vi "Email Handler (PC).vi"() -> ()   [LabVIEW 2019]
uses:
  Controls/Alarm Config.ctl
  Controls/Alarm Definition.ctl
  Controls/Alarm Profile Config.ctl
panel:
  in  "Boolean":bool
  out "Tab Control":enum32{"Page 1", "Page 2"}(tab)
  in  "Email To:":string
  out "Unsent Emails":i32
  in  "Script Path":path=path "C:/Projects/Alarm Email Handler/Executable/Script/gmail_script.py"
  in  "Path to Python.exe":path=path "C:/Python35-32/python.exe"
  # "Keep Running\nand Minimized"
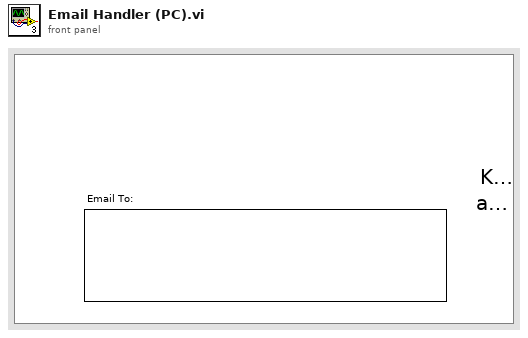
[diagram p1: front panel]
types:
  T1 = cluster{"ArmedAddresses":i32[], "Tracker":i32, "Armed":bool, "Email To:":string, "Alarm":bool, "Unsent Emails":i32, "IP to Check":i32, "Email Data":string[], "Email Config Path":path}
  T2 = enum16{"open", "replace", "create", "open or create", "replace or create", "replace or create with confirmation"}
  T3 = typedef "Alarm Config.ctl" = cluster{"Alarms:":T4[], "Profile Sync:":T5}
  T4 = typedef "Alarm Definition.ctl" = cluster{"Description:":string, "Enabled:":bool, "Data Index:":i32, "Data Type:":string, "Low Limit:":dbl, "High Limit:":dbl, "Trip Time:":u32, "Profile Sync:":bool}
  T5 = typedef "Alarm Profile Config.ctl" = cluster{"Trip Time:":u32, "Consecutive Trips:":i32}
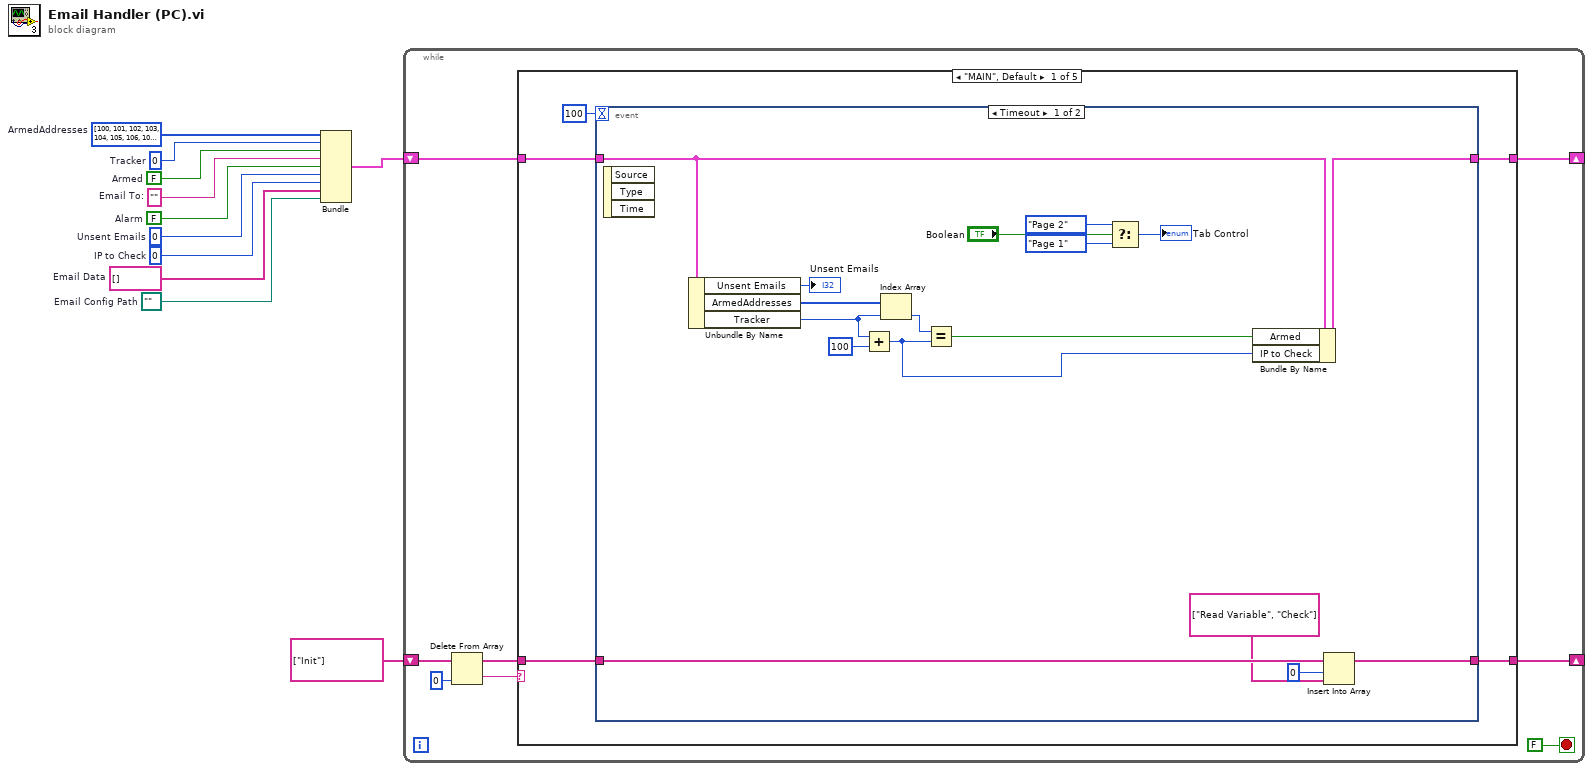
[diagram p0: block diagram]
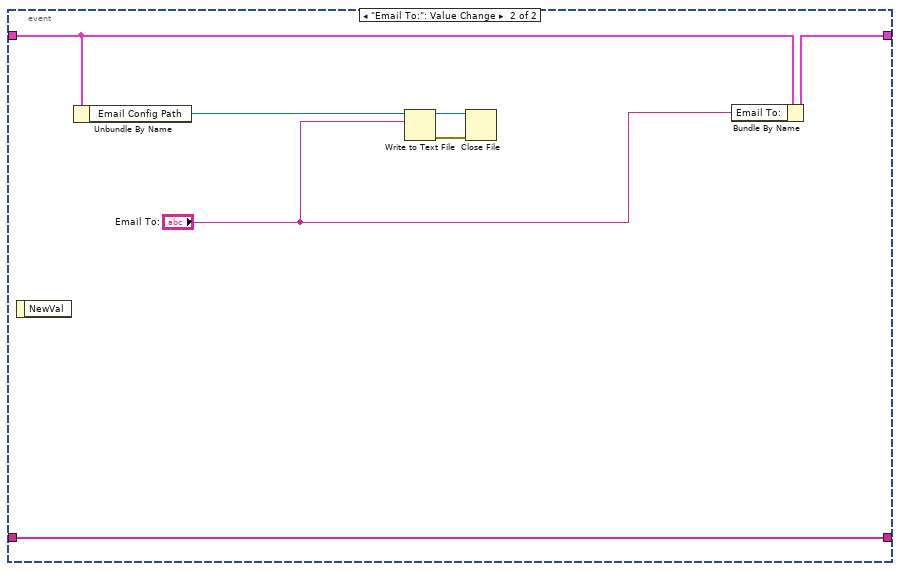
[diagram p2: hidden frame]
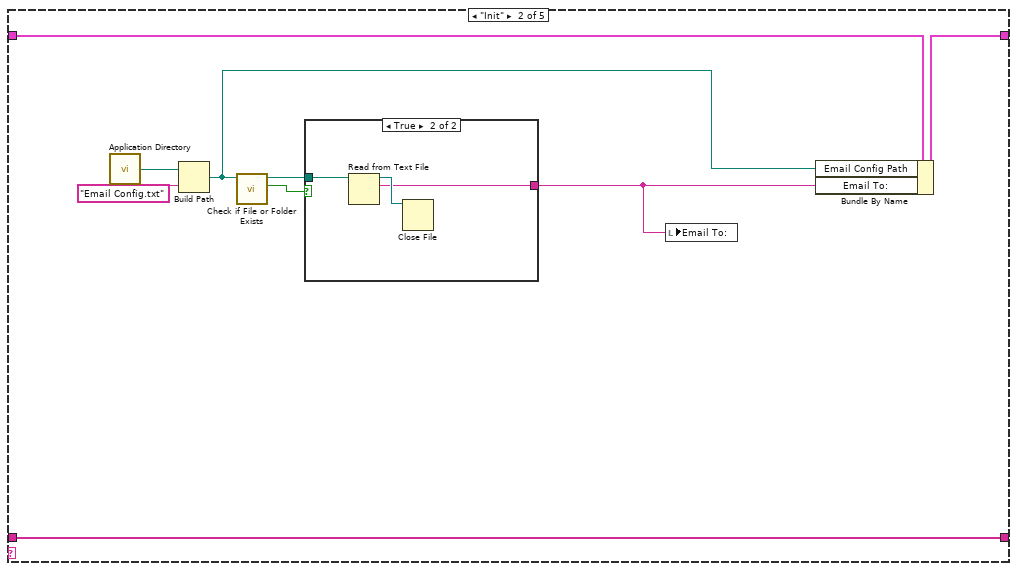
[diagram p3: hidden frame]
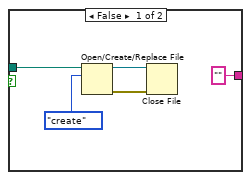
[diagram p4: hidden frame]
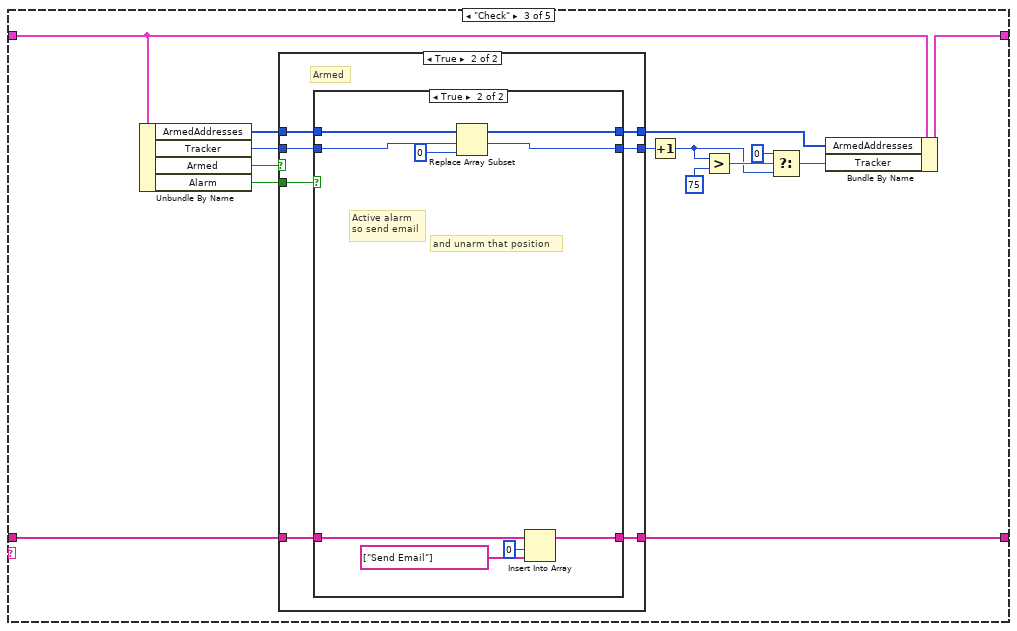
[diagram p5: hidden frame]
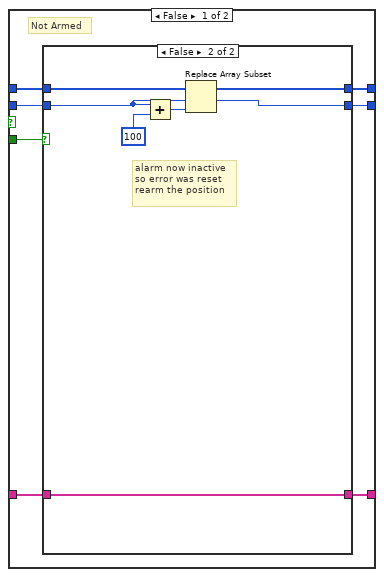
[diagram p6: hidden frame]
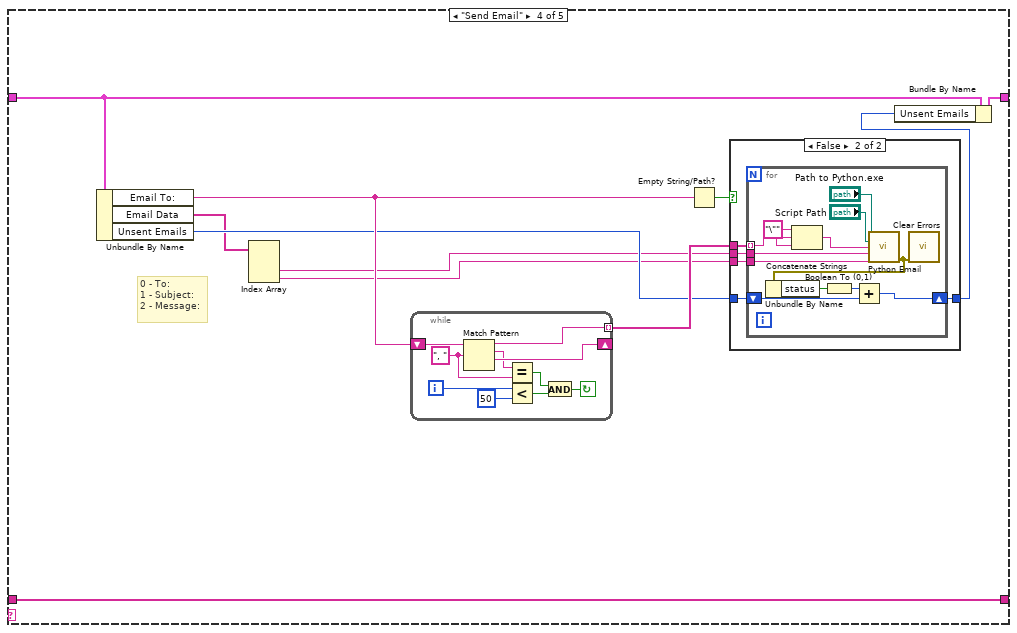
[diagram p9: hidden frame]
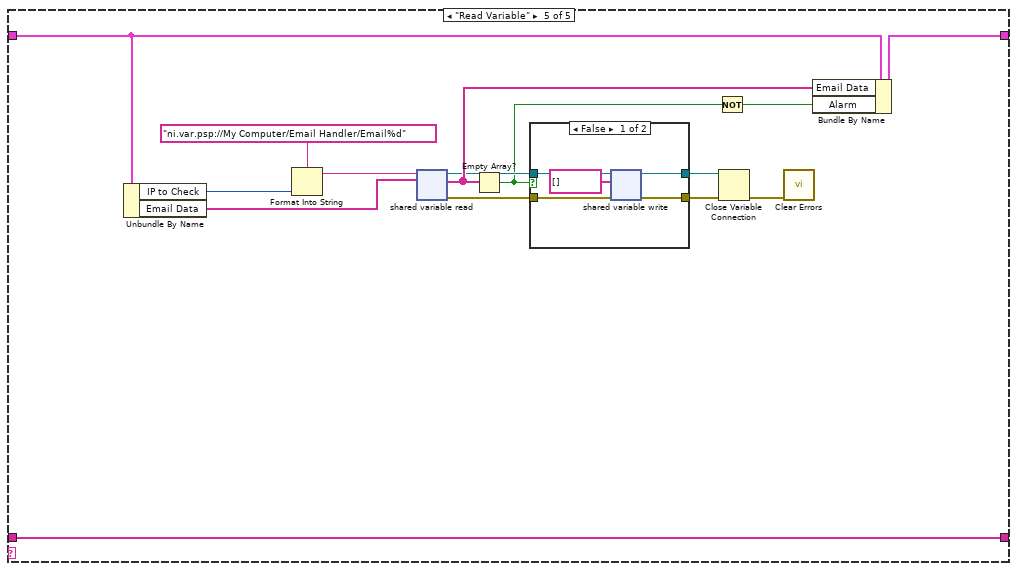
[diagram p11: hidden frame]
diagram:
  w1 = path ""  # Email Config Path
  w2 = string[] []  # Email Data
  w3 = 0  # IP to Check
  w4 = 0  # Unsent Emails
  w5 = FALSE  # Alarm
  w6 = ""  # Email To:
  w7 = FALSE  # Armed
  w9 = i32[] [100, 101, 102, 103, 104, 105, 106, 107, 108, 109, 110, 111, 112, 113, 114, 115, 116, 117, 118, 119, 120, 121, 122, 123, 124, 125, 126, 127, 128, 129, 130, 131, 132, 133, 134, 135, 136, 137, 138, 139, 140, 141, 142, 143, 144, 145, 146, 147, 148, 149, 150, 151, 152, 153, 154, 155, 156, 157, 158, 159, 160, 161, 162, 163, 164, 165, 166, 167, 168, 169, 170, 171, 172, 173, 174, 175]  # ArmedAddresses
  w11 = 0  # Tracker
  n1 = Bundle("ArmedAddresses"=w9, "Tracker"=w11, "Armed"=w7, "Email To:"=w6, "Alarm"=w5, "Unsent Emails"=w4, "IP to Check"=w3, "Email Data"=w2, "Email Config Path"=w1) -> (w10:T1)  [unwired: 1 in]
  n2 = while {
    shift-right: [w12] -> _
    shift-left: w10 -> [w18]
    shift-right: [w13] -> _
    shift-left: string[] ["Init"] -> [w17]
    stop <- FALSE stop-if-true
    n3 = Delete From Array(array=w17, index=0) -> (deleted portion=w15:string, array with subset deleted=w14:string[])  [unwired: 1 in]
    n4 = case shown="\"MAIN\", Default" w15 {
      tunnel: w18 -> [w24 w52 w75 w120 w166]
      tunnel: w14 -> [w22 w57 w72 w125 w168]
      tunnel: [w21 w57 w69 w125 w168] -> w13
      tunnel: [w23 w51 w74 w119 w167] -> w12
      frame "MAIN", Default {
        n5 = event shown="[0] Timeout" {
          selector: _ -> [_ _]
          dyn-events: _ -> [_ _]
          timeout: 100 -> [_ _]
          tunnel: w24 -> [w40 w47]
          tunnel: [w39 w46] -> w23
          tunnel: w22 -> [w35 w48]
          tunnel: [w25 w48] -> w21
          event Timeout {
            n6 = event-data() -> ()  [unwired: 1 in, 3 out]
            n7 = Unbundle By Name(w40) -> ("Unsent Emails"=→"Unsent Emails":i32, "ArmedAddresses"=w41:i32[], "Tracker"=w32:i32)
            n8 = Add(x=w32, y=100) -> (x+y=w26:i32)
            n9 = Index Array(array=w41, index=w32) -> (element=w37:i32)
            n10 = Equal?(x=w37, y=w26) -> (x = y?=w36:bool)
            n11 = Select(t=enum32{"Page 1", "Page 2"}."Page 2" ("Tab Control"), s="Boolean", f=enum32{"Page 1", "Page 2"}."Page 1" ("Tab Control")) -> (s? t:f=→"Tab Control":enum32{"Page 1", "Page 2"})
            n12 = Bundle By Name(cluster=w40, "Armed"=w36, "IP to Check"=w26) -> (w39:T1)
            n13 = Insert Into Array(array=w35, index=0, new element=string[] ["Read Variable", "Check"]) -> (w25:string[])
          }
          event "Email To:": Value Change {
            n14 = event-data() -> ()  [unwired: 1 in, 1 out]
            n15 = Unbundle By Name(w47) -> ("Email Config Path"=w45:path)
            n16 = Write to Text File(file (use dialog)=w45, text="Email To:") -> (refnum out=w44:refnum<file>, error out=w43:errorcluster)  [unwired: 2 in, 1 out]
            n17 = Close File(refnum=w44, error in=w43) -> ()  [unwired: 2 out]
            n18 = Bundle By Name(cluster=w47, "Email To:"="Email To:") -> (w46:T1)
          }
        }
      }
      frame "Init" {
        n19 = call <vilib>:"Application Directory.vi"() -> ("Application Directory"=w54:path)
        n20 = Build Path(base path=w54, name or relative path="Email Config.txt") -> (appended path=w50:path)
        n21 = call <vilib>:"Check if File or Folder Exists.vi"("path"=w50) -> ("file or folder exists?"=w55:bool, "dup path"=w56:path)  [unwired: 8 in, 1 out]
        n22 = case shown="True" w55 {
          tunnel: w56 -> [w61 w65]
          tunnel: ["" w63] -> w49
          frame False {
            (unwired) T3 {"Alarms:"=[{"Description:"="", "Enabled:"=FALSE, "Data Index:"=0, "Data Type:"="", "Low Limit:"=0.0, "High Limit:"=0.0, "Trip Time:"=0, "Profile Sync:"=FALSE}, {"Description:"="", "Enabled:"=FALSE, "Data Index:"=0, "Data Type:"="", "Low Limit:"=0.0, "High Limit:"=0.0, "Trip Time:"=0, "Profile Sync:"=FALSE}, {"Description:"="", "Enabled:"=FALSE, "Data Index:"=0, "Data Type:"="", "Low Limit:"=0.0, "High Limit:"=0.0, "Trip Time:"=0, "Profile Sync:"=FALSE}, {"Description:"="", "Enabled:"=FALSE, "Data Index:"=0, "Data Type:"="", "Low Limit:"=0.0, "High Limit:"=0.0, "Trip Time:"=0, "Profile Sync:"=FALSE}, {"Description:"="", "Enabled:"=FALSE, "Data Index:"=0, "Data Type:"="", "Low Limit:"=0.0, "High Limit:"=0.0, "Trip Time:"=0, "Profile Sync:"=FALSE}, {"Description:"="", "Enabled:"=FALSE, "Data Index:"=0, "Data Type:"="", "Low Limit:"=0.0, "High Limit:"=0.0, "Trip Time:"=0, "Profile Sync:"=FALSE}, {"Description:"="", "Enabled:"=FALSE, "Data Index:"=0, "Data Type:"="", "Low Limit:"=0.0, "High Limit:"=0.0, "Trip Time:"=0, "Profile Sync:"=FALSE}, {"Description:"="", "Enabled:"=FALSE, "Data Index:"=0, "Data Type:"="", "Low Limit:"=0.0, "High Limit:"=0.0, "Trip Time:"=0, "Profile Sync:"=FALSE}], "Profile Sync:"={"Trip Time:"=0, "Consecutive Trips:"=0}} ("Alarm Config")
            n23 = Open/Create/Replace File(file path (use dialog)=w61, operation (0:open)=T2."create") -> (refnum out=w60:refnum<file>, error out=w59:errorcluster)  [unwired: 4 in, 1 out]
            n24 = Close File(refnum=w60, error in=w59) -> ()  [unwired: 2 out]
          }
          frame True {
            n25 = Read from Text File(file (use dialog)=w65) -> (refnum out=w64:refnum<file>, text=w63:string)  [unwired: 3 in, 2 out]
            n26 = Close File(refnum=w64) -> ()  [unwired: 1 in, 2 out]
          }
        }
        n27 = local write "Email To:"(w49) -> ()
        n28 = Bundle By Name(cluster=w52, "Email Config Path"=w50, "Email To:"=w49) -> (w51:T1)
      }
      frame "Check" {
        n29 = Unbundle By Name(w75) -> ("ArmedAddresses"=w68:i32[], "Tracker"=w71:i32, "Armed"=w73:bool, "Alarm"=w66:bool)
        n30 = case shown="True" w73 {
          tunnel: w72 -> [w87 w103]
          tunnel: w71 -> [w84 w100]
          tunnel: [w81 w97] -> w70
          tunnel: w66 -> [w83 w101]
          tunnel: [w86 w102] -> w69
          tunnel: w68 -> [w85 w99]
          tunnel: [w82 w98] -> w67
          frame False {
            # "Not Armed"
            n31 = case shown="False" w83 {
              tunnel: w87 -> [w88 w91]
              tunnel: [w88 w91] -> w86
              tunnel: w84 -> [w89 w94]
              tunnel: w85 -> [w90 w96]
              tunnel: [w90 w95] -> w82
              tunnel: [w89 w94] -> w81
              frame True {
                # "Alarm still active\nerror has not been reset\nleave unarmed"
              }
              frame False {
                # "alarm now inactive\nso error was reset\nrearm the position"
                n32 = Add(x=w94, y=100) -> (x+y=w93:i32)
                n33 = Replace Array Subset(array=w96, new element=w93, index=w94) -> (w95:i32[])
              }
            }
          }
          frame True {
            # "Armed"
            n34 = case shown="True" w101 {
              tunnel: w103 -> [w104 w114]
              tunnel: [w104 w113] -> w102
              tunnel: w100 -> [w105 w108]
              tunnel: w99 -> [w106 w110]
              tunnel: [w106 w109] -> w98
              tunnel: [w105 w108] -> w97
              frame False {
                # "No Alarm"
              }
              frame True {
                # "and unarm that position"
                # "Active alarm\nso send email"
                n35 = Replace Array Subset(array=w110, new element=0, index=w108) -> (w109:i32[])
                n36 = Insert Into Array(array=w114, index=0, new element=string[] ["Send Email"]) -> (w113:string[])
              }
            }
          }
        }
        n37 = Increment(x=w70) -> (x+1=w77:i32)
        n38 = Greater?(x=w77, y=75) -> (0:w79:bool)
        n39 = Select(t=0, s=w79, f=w77) -> (s? t:f=w76:i32)
        n40 = Bundle By Name(cluster=w75, "ArmedAddresses"=w67, "Tracker"=w76) -> (w74:T1)
      }
      frame "Send Email" {
        # "0 - To:\n1 - Subject:\n2 - Message:"
        n41 = Unbundle By Name(w120) -> ("Email To:"=w123:string, "Email Data"=w117:string[], "Unsent Emails"=w121:i32)
        n42 = Index Array(array=w117) -> (element #2=w116:string, element #3=w115:string)  [unwired: 3 in, 1 out]
        n43 = while {
          shift-right: [w134] -> _
          shift-left: w123 -> [w135]
          tunnel: [w131] -> w122 mode=indexing
          i -> [w130]
          stop <- w126 continue-if-true
          w132 = ", " ("search string")
          n44 = Match Pattern(string=w135, regular expression=w132) -> (before substring=w131:string, match substring=w133:string, after substring=w134:string)  [unwired: 1 in, 1 out]
          n45 = Equal?(x=w133, y=w132) -> (x = y?=w127:bool)
          n46 = Less?(x=w130, y=50) -> (x < y?=w128:bool)
          n47 = And(x=w127, y=w128) -> (x .and. y?=w126:bool)
        }
        n48 = Empty String/Path?(string/path=w123) -> (empty?=w124:bool)
        n49 = case shown="False" w124 {
          tunnel: w115 -> [_ w139]
          tunnel: w116 -> [_ w140]
          tunnel: w122 -> [_ w141]
          tunnel: w121 -> [w136 w138]
          tunnel: [w136 w137] -> w118
          frame True {
          }
          frame False {
            n50 = for {
              tunnel: w141 -> [w150] mode=indexing
              tunnel: w140 -> [w153]
              tunnel: w139 -> [w152]
              shift-right: [w145] -> w137
              shift-left: w138 -> [w147]
              w151 = "\"" ("string")
              n51 = Concatenate Strings(w151, w150, w151) -> (w149:string)
              n52 = call "Python Email.vi"("Path to Python.exe"="Path to Python.exe", "Script Path"="Script Path", "To:"=w149, "Subject:"=w153, "Message:"=w152) -> ("error out"=w144:errorcluster)  [unwired: 6 in, 4 out]
              n53 = Unbundle By Name(w144) -> ("status"=w148:bool)
              n54 = Boolean To (0,1)(Boolean=w148) -> (0, 1=w146:i16)
              n55 = Add(x=w146, y=w147) -> (x+y=w145:i32)
              n56 = call <vilib>:"Clear Errors.vi"("error in (no error)"=w144) -> ()  [unwired: 5 in, 2 out]
            }
          }
        }
        n57 = Bundle By Name(cluster=w120, "Unsent Emails"=w118) -> (w119:T1)
      }
      frame "Read Variable" {
        n58 = Unbundle By Name(w166) -> ("IP to Check"=w164:i32, "Email Data"=w162:string[])
        n59 = Format Into String(format string="ni.var.psp://My Computer/Email Handler/Email%d", w164) -> (resulting string=w163:string)  [unwired: 2 in, 1 out]
        n60 = shared-variable-read(w163, w162) -> (w160:refnum<k21>, w159:errorcluster, w161:string[])  [unwired: 1 in, 1 out]
        n61 = Empty Array?(array=w161) -> (empty?=w156:bool)
        n62 = case shown="False" w156 {
          tunnel: w160 -> [w173 w175]
          tunnel: w159 -> [w172 w174]
          tunnel: [w170 w175] -> w158
          tunnel: [w169 w174] -> w157
          frame False {
            n63 = shared-variable-write(w173, w172, string[] [] ("data in")) -> (w170:refnum<k21>, w169:errorcluster)
          }
          frame True {
          }
        }
        n64 = Not(x=w156) -> (.not. x?=w154:bool)
        n65 = Close Variable Connection(8:w157, 11:w158) -> (0:w155:errorcluster)
        n66 = call <vilib>:"Clear Errors.vi"("error in (no error)"=w155) -> ()  [unwired: 5 in, 2 out]
        n67 = Bundle By Name(cluster=w166, "Email Data"=w161, "Alarm"=w154) -> (w167:T1)
      }
    }
  }
